vi "Execute Lua Script.vi"(4 "nresults":i32=-1, 6 "nargs":i32=-1, 8 "error in (no error)":errorcluster, 10 "lua script":string, 11 "Lua in":refnum<data-value>) -> (0 "error out":errorcluster, 3 "Lua out":refnum<data-value>)   [LabVIEW 2020, in "Lua for LabVIEW.lvlib" / "Lua.lvclass"]
doc: "Load and execute a Lua script. Specify the number of return values expected from the script using the nresults argument. For example, to return a number from a script, the script could end with:\n\n...\nreturn my_number_result\n\nIf nargs = -1, then any values on the stack at the time of the call will be passed to the script.\nIf nresult = -1, then all values returned from the script will be left on the stack after the call."
uses:
  Lua.lvclass
  Lua.lvclass/Lua.ctl
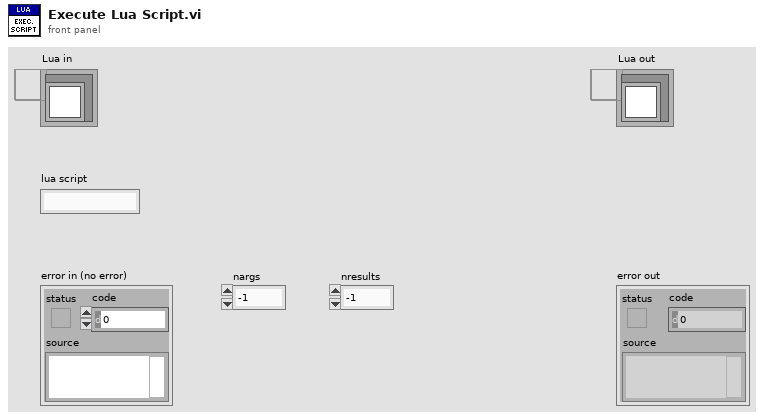
[diagram p1: front panel]
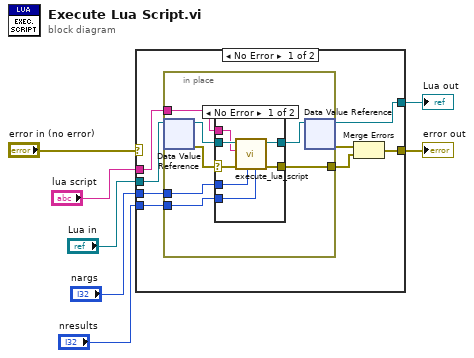
[diagram p0: block diagram]
diagram:
  n1 = case shown="No Error" "error in (no error)" {
    selector: "error in (no error)" -> [_ w33]
    tunnel: [w13 w33] -> w6
    tunnel: [w11 w32] -> w4
    tunnel: "Lua in" -> [w15 w32]
    tunnel: "lua script" -> [w10 _]
    tunnel: "nargs" -> [w9 _]
    tunnel: "nresults" -> [w8 _]
    frame No Error {
      n2 = in-place {
        in-place-border: [w19] -> w12
        in-place-border: w10 -> [w18]
        in-place-border: w9 -> [w17]
        in-place-border: w8 -> [w16]
        n3 = in-place-dvr #1(w15) -> (w22:refnum<class "Lua.lvclass">, w20:errorcluster)
        n4 = case shown="No Error" w20 {
          selector: w20 -> [w26 w31]
          tunnel: w22 -> [w29 w30]
          tunnel: [w28 w30] -> w21
          tunnel: [w27 w31] -> w19
          tunnel: w18 -> [w25 _]
          tunnel: w17 -> [w24 _]
          tunnel: w16 -> [w23 _]
          frame No Error {
            n5 = call-dynamic "execute_lua_script.vi"("nresults"=w23, "nargs"=w24, "error in (no error)"=w26, "lua script"=w25, "Lua in"=w29) -> ("error out"=w27:errorcluster, "Lua out"=w28:refnum<class "Lua.lvclass">)  [unwired: 5 in]
          }
          frame Error {
          }
        }
        n6 = in-place-dvr #1(w21) -> (w11:refnum<data-value>, w14:errorcluster)
      }
      n7 = Merge Errors(w14, w12) -> (w13:errorcluster)
    }
    frame Error {
    }
  }
  "error out" <- w6
  "Lua out" <- w4
